vi "Udp Tester 3.vi"() -> ()   [LabVIEW 2014]
uses:
  <vilib>/addons/control/pid/pid.llb/PID EGU to Percentage (DBL).vi
  <vilib>/addons/control/pid/autopid.llb/PID Online Autotuning (Relay Feedback).vi
  <vilib>/addons/control/pid/pid.llb/PID Percentage to EGU (DBL).vi
  <vilib>/addons/control/pid/pid.llb/PID Advanced (DBL).vi
  <vilib>/FPGAPlugInAG/myRIO-1900/niLvFpga_Open_myRIO-1900.vi
  <vilib>/rvi/interface/common/dynamic/niFpgaDynamicAddResources.vi
  <vilib>/Utility/error.llb/Error Cluster From Error Code.vi
  <vilib>/rvi/errors/niLvFpgaAdjustHostInterfaceError.vi
  <vilib>/Utility/file.llb/Write To Spreadsheet File (I64).vi
  <vilib>/FPGAPlugInAG/Dynamic/niLvFpga_Close_Dynamic.vi
  <vilib>/rvi/interface/nirviOpenFPGA/nirviOpenFPGA.xnode
  FPGA Bitfiles/Test_FPGATarget_CurrentControl_60eBuCSPTsI.lvbitx
  Current Control.vi
  <vilib>/rvi/interface/nirviReadWriteControl/nirviReadWriteControl.xnode
  <vilib>/rvi/interface/nirviCloseFPGA/nirviCloseFPGA.xnode
  <vilib>/rvi/interface/Simulation/niFpgaSimulationCallBeginRW.vi
  NiFpgaLv.dll
  <vilib>/addons/control/pid/NI_PID_autopid.lvlib
  <vilib>/addons/control/pid/NI_PID_pid.lvlib
panel:
  in  "Final Output Unit":enum16{"%", "EGU"}(ring)=enum."EGU"
  in  "PID Final Min":dbl format="%.2f"
  in  "PID Final Max":dbl format="%.2f"
  in  "Intermediate Output Unit":enum16{"%", "EGU"}(ring)=enum."EGU"
  in  "Max Out":dbl format="%.2f"
  in  "Min Out":dbl format="%.2f"
  in  "Input Unit":enum16{"%", "EGU"}(ring)
  out "MV":dbl(graph)=20.39115328927357
  in  "Tab Control":enum32{"Instructions", "Plant Parameters"}(tab)
  in  "Instructions":string="Overview: This example demonstrates how to use the  PID Online Autotuning VI with the PID using the Relay Autotuning Technique.\nInstructions:\n1. Run the VI and wait until the process variable (PV) reaches near setpoint (SP).\n2.  On the PID Autotuning Design section, select the type of algorithm, type of controller and excitation amplitude for the 'open loop step response'. Then, click Autotune to start the process.\n3.  When the tuned PID gains do not change anymore or the tuning completed? flashes, the identification is done and you can accept new gains by pressing Accept gain and that will transfer the new gain to PID Gains.\n4. Click Autotune again to go back to the automatic control. You can try different options and repeat this process.\n5. Click Stop to stop the VI.\n"
  out "Plant Variable Gain":dbl=5.68817109595442
  out "Plant Variable Lag":dbl=1.4596237458843302
  in  "Load":dbl(slide) scale=0.0..10.0
  in  "Stop":bool
  out "SP and PV":cluster{"Plant Output":dbl, "SP:":dbl}(graph)
  in  "Sampling Time dt (s)":dbl=0.05 min=0.001 step=0.01 format="%#.3p"
  in  "PID Gains":T1={"proportional gain (Kc)"=0.05, "integral time (Ti, min)"=0.0, "derivative time (Td, min)"=0.0} {"derivative time (Td, min)" format="%#.6g"; "integral time (Ti, min)" format="%#.6g"; "proportional gain (Kc)" format="%#.6g"}
  in  "SP:":dbl(slide)=28.758169934640524 min=0.0 max=0.0 scale=400.0..750.0
  out "PV:":dbl(slide)=28.4408554797721 scale=400.0..750.0
  in  "Autotune":bool
  in  "Accept gain":bool
  out "tuned PID gains":T1={"proportional gain (Kc)"=1.9838195929127882, "integral time (Ti, min)"=0.01995856284686879, "derivative time (Td, min)"=0.0} {"derivative time (Td, min)" format="%#.6g"; "integral time (Ti, min)" format="%#.6g"; "proportional gain (Kc)" format="%#.6g"}
  in  "autotuning parameters":T2={"Type of Controller"=0, "relay cycles"=3, "relay amplitude"=1.0, "control specifications"=2, "PV noise level"=0.1} {"PV noise level" format="%.2f"; "control specifications" items=["fast", "normal", "slow"]; "relay amplitude" format="%.2f"; "Type of Controller" items=["P", "PI", "PID"]}
  in  "Reinitialize":bool
  in  "Automatic":bool=TRUE
  in  "alpha":dbl(slide)=0.49999999999999994 scale=0.0..1.0
  out "tuning completed?":bool
  in  "gamma":dbl(slide)=0.5102040816326531 scale=0.0..1.0
  in  "MV":dbl=60.0 format="%#_13g"
  out "error out":errorcluster
  out "Status?":bool
  out "Head Position":i32
  # "Plant Simulated Parameters"
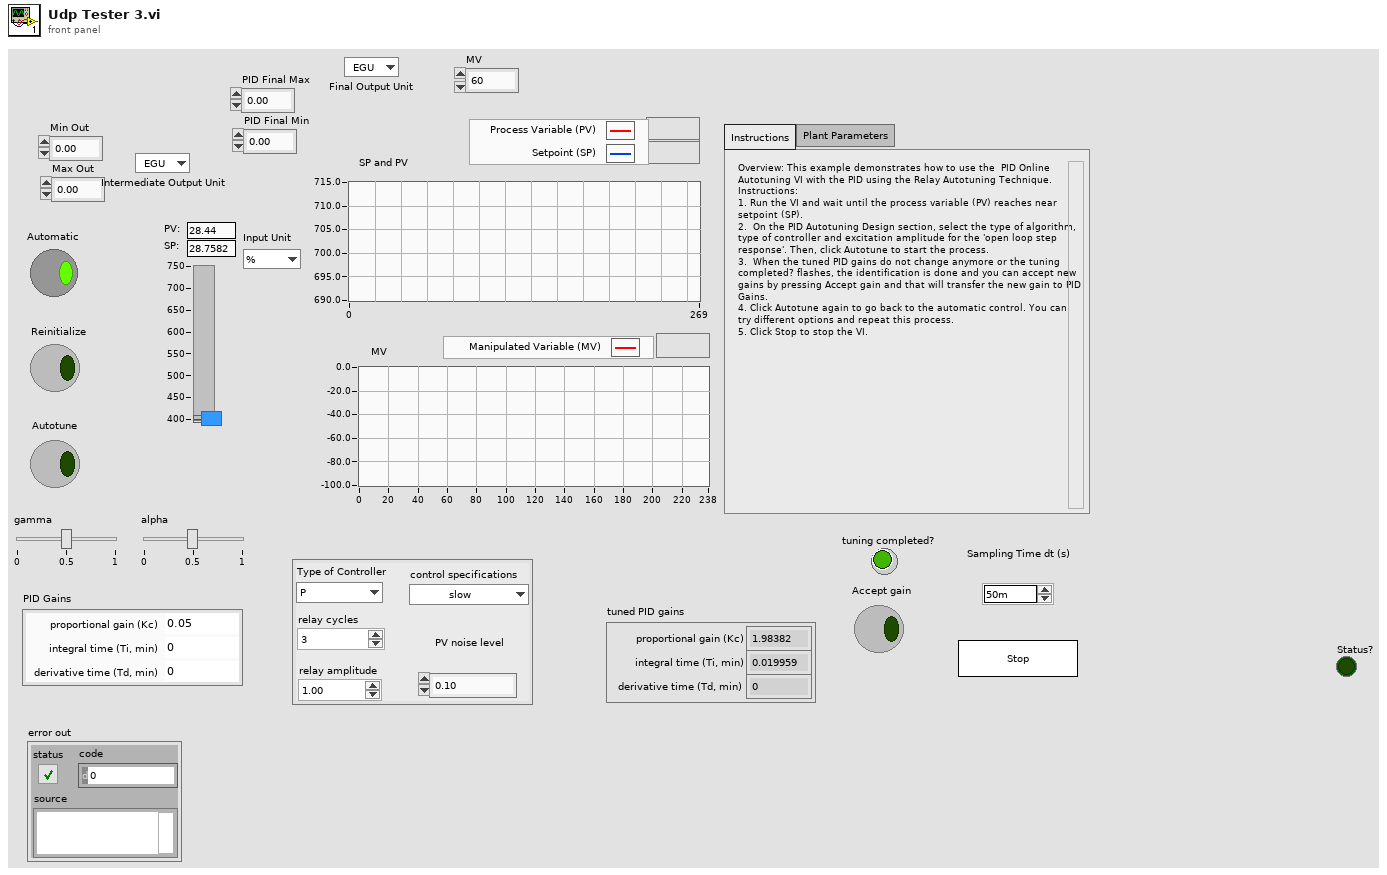
[diagram p1: front panel]
types:
  T1 = cluster{"proportional gain (Kc)":dbl, "integral time (Ti, min)":dbl, "derivative time (Td, min)":dbl}
  T2 = cluster{"Type of Controller":u16, "relay cycles":i32, "relay amplitude":dbl, "control specifications":u16, "PV noise level":dbl}
  T3 = cluster{"static gain":dbl, "lag (s)":dbl, "deadtime (s)":dbl, "load":dbl, "deadband":dbl, "sensor noise":dbl, "initial PV":dbl, "plant noise":dbl}
  T4 = enum16{"big-endian, network order", "native, host order", "little-endian"}
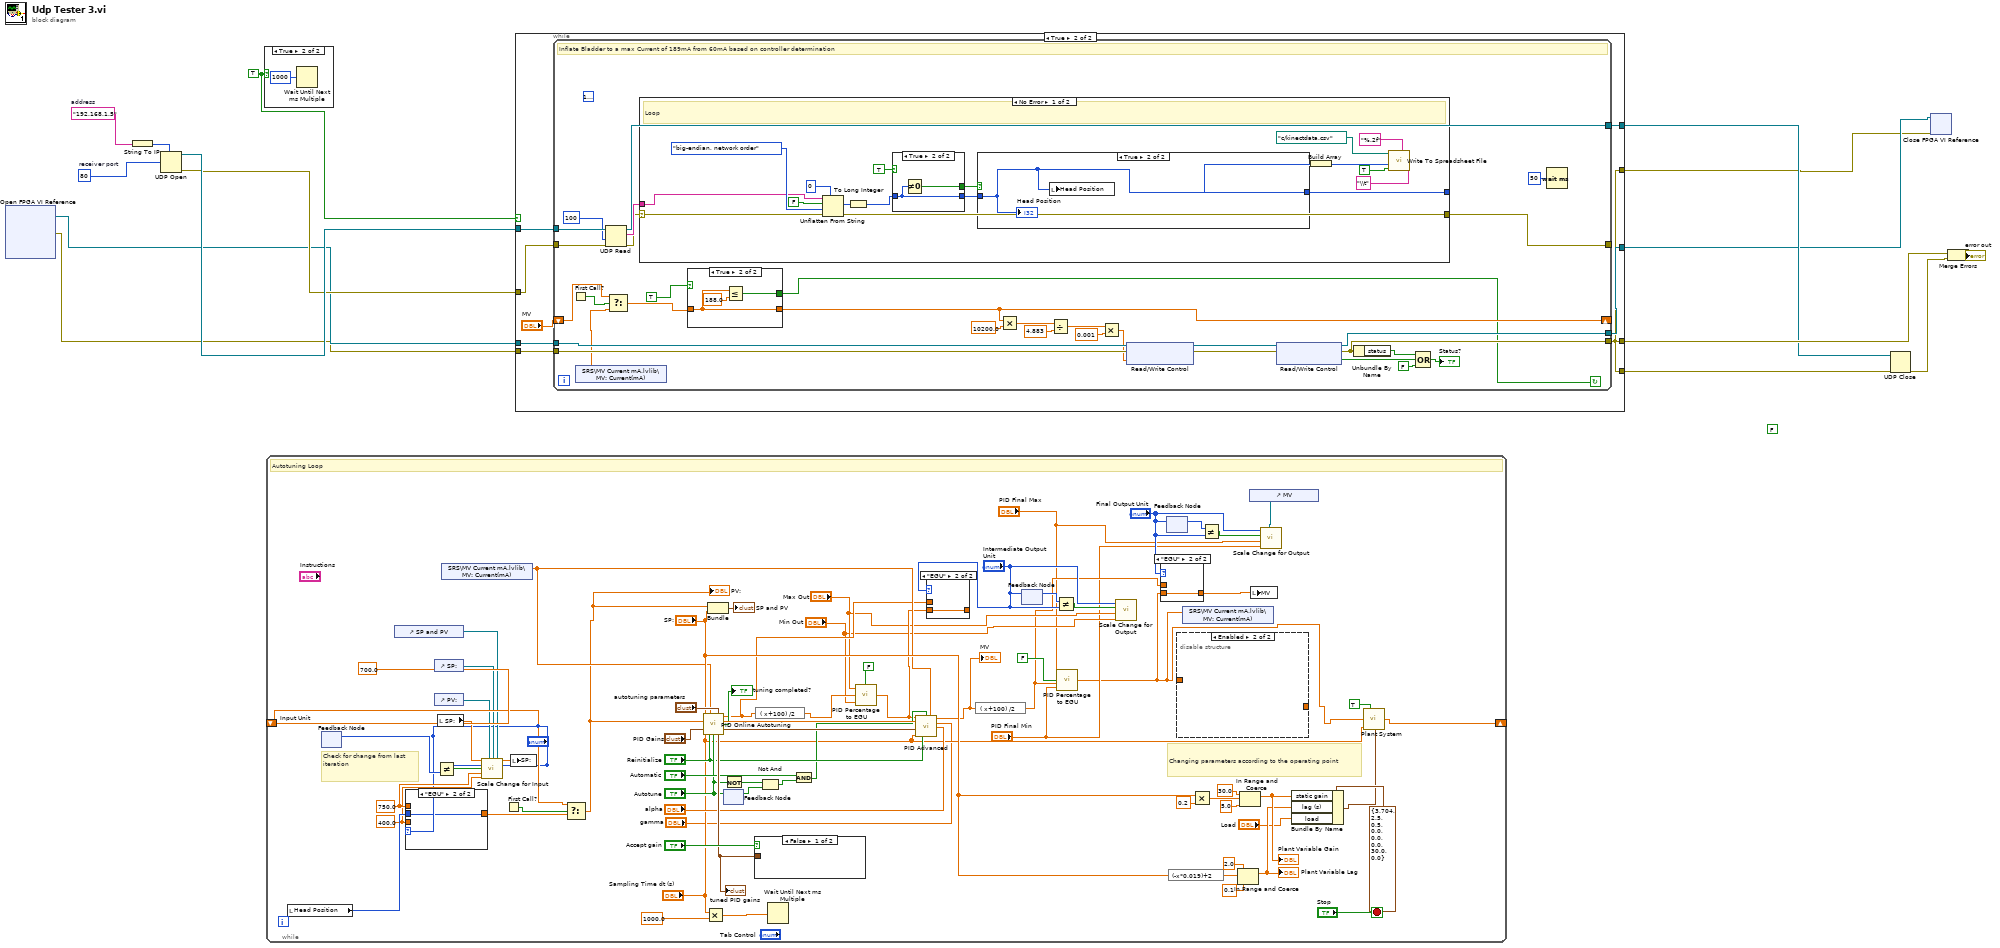
[diagram p0: block diagram]
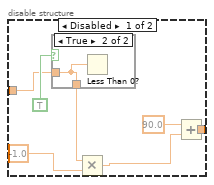
[diagram p2: hidden frame]
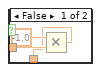
[diagram p3: hidden frame]
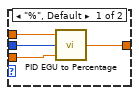
[diagram p6: hidden frame]
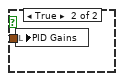
[diagram p7: hidden frame]
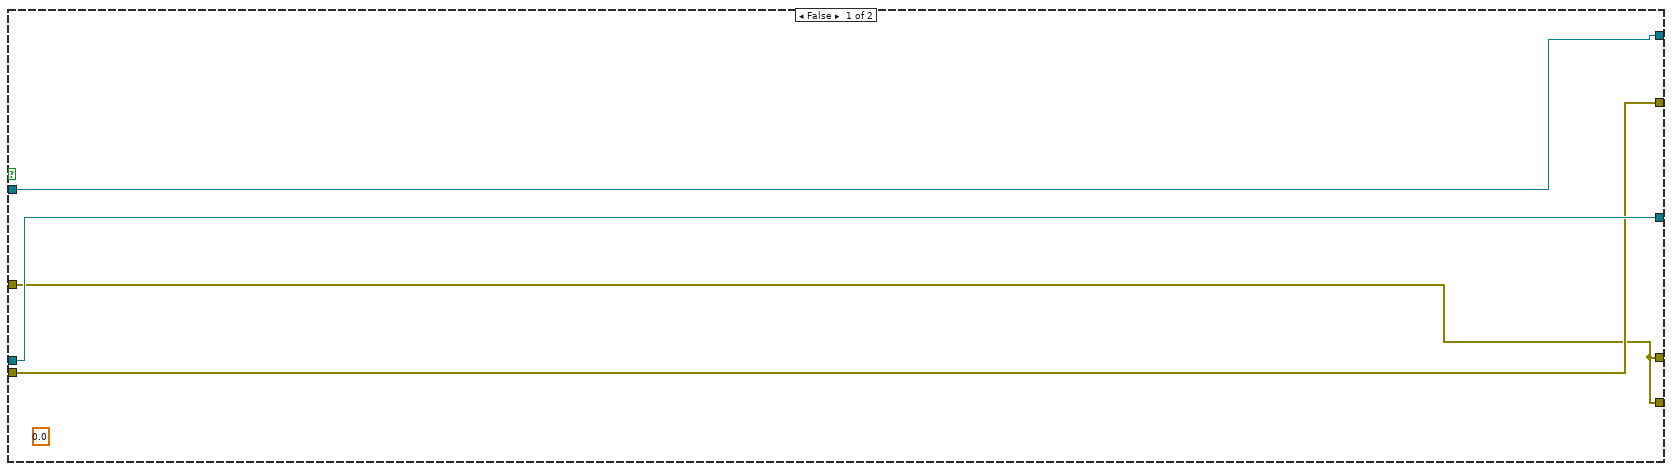
[diagram p9: hidden frame]
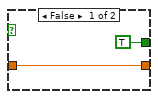
[diagram p10: hidden frame]
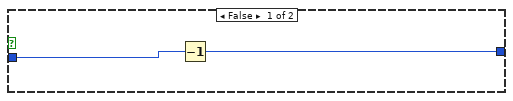
[diagram p11: hidden frame]
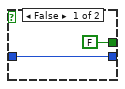
[diagram p12: hidden frame]
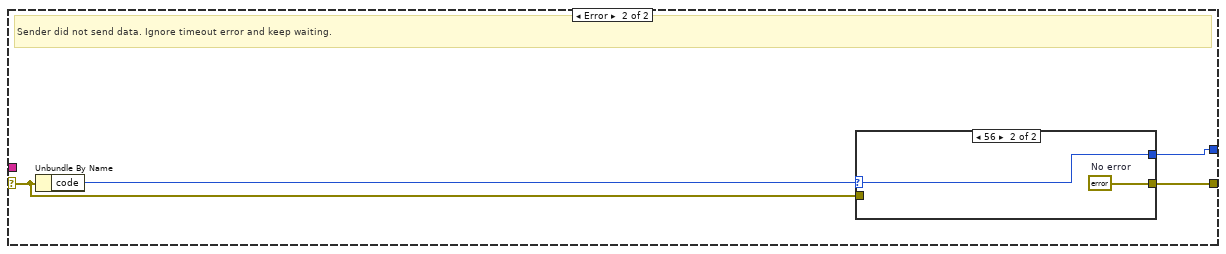
[diagram p13: hidden frame]
diagram:
  w2 = TRUE
  (unwired) FALSE
  w15 = "192.168.1.5"  # address
  w14 = u16 80  # receiver port
  n1 = xnode "Open FPGA VI Reference"() -> ("FPGA VI Reference Out"=w4:refnum<k20>, "error out"=w3:errorcluster)  [unwired: 2 in]
  n2 = String To IP(1:w15) -> (0:w16:u32)
  n3 = UDP Open(7:w16, 11:w14) -> (port=w13:refnum<k16>, 0:w12:errorcluster)  [unwired: 3 in, 1 out]
  n4 = case shown="True" w2 {
    frame False {
    }
    frame True {
      n5 = Wait Until Next ms Multiple(millisecond multiple=u32 1000) -> ()  [unwired: 1 out]
    }
  }
  n6 = while {
    shift-left: 700.0 ("Plant Output") -> [w51]
    shift-right: [w87] -> _
    stop <- "Stop" stop-if-true
    w45 = 750.0 ("Max In")
    w44 = 400.0 ("Min In")
    # "Check for change from last iteration"
    # "Changing parameters according to the operating point"
    # "Autotuning Loop"
    n7 = local read "Head Position"() -> (w49:i32)
    n8 = feedback #1() -> (w47:enum16{"%", "EGU"})  [unwired: 1 out]
    n9 = feedback-in #1("Input Unit") -> ()
    n10 = control-ref of="SP and PV"() -> (w40:refnum<vi>)
    n11 = case shown="\"EGU\"" "Input Unit" {
      tunnel: w49 -> [w108 w109]
      tunnel: [w107 w109] -> w48
      tunnel: w45 -> [w106 _]
      tunnel: w44 -> [w105 _]
      frame "%", Default {
        n12 = call-poly <vilib>:"PID EGU to Percentage.vi"("minimum (EGU)"=w105, "input (EGU)"=w108, "maximum (EGU)"=w106) -> ("% span"=w107:dbl)
      }
      frame "EGU" {
      }
    }
    n13 = control-ref of="SP:"() -> (w39:refnum<vi>)
    n14 = control-ref of="PV:"() -> (w41:refnum<vi>)
    n15 = Not Equal?(x="Input Unit", y=w47) -> (x != y?=w46:bool)
    n16 = local read "SP:"() -> (w42:dbl)
    n17 = shared-variable "SRS\\MV Current mA.lvlib\\MV: Current(mA)"() -> (w53:dbl)  [unwired: 1 in, 1 out]
    n18 = call "Scale Change for Input.vi"("SP:"=w42, "Slide Refnum"=w41, "Slide Refnum 2"=w39, "WFChart Refnum"=w40, "Input Unit"="Input Unit", "Change Scales"=w46, "Max In"=w45, "Min In"=w44) -> ("SP After Scale Change"=w43:dbl)  [unwired: 3 in, 4 out]
    n19 = First Call?() -> (First Call?: T/F=w52:bool)
    n20 = local write "SP:"(w43) -> ()
    n21 = Select(t=w51, s=w52, f=w48) -> (s? t:f=w50:dbl)
    "PV:" <- w50
    n22 = call-poly <vilib>:"PID Online Autotuning.vi"("setpoint"="SP:", "manipulated variable"=w53, "autotuning parameters"="autotuning parameters", "process variable"=w50, "PID gains in"="PID Gains", "dt (s)"="Sampling Time dt (s)", "reinitialize? (F)"="Reinitialize", "autotune? (F)"="Autotune") -> ("setpoint out"=w35:dbl, "process variable out"=w78:dbl, "tuning completed?"=→"tuning completed?":bool, "PID gains out"=w74:T1, "tuned PID gains"=w73:T1)  [unwired: 3 in]
    "tuned PID gains" <- w73
    n23 = Multiply(x="Sampling Time dt (s)", y=1000.0) -> (x*y=w55:dbl)
    n24 = Bundle("% span"=w50, "SP:"="SP:") -> (→"SP and PV":cluster{"% span":dbl, "SP:":dbl})  [unwired: 1 in]
    n25 = feedback #2() -> (w71:bool)  [unwired: 1 in]
    n26 = feedback-in #2("Autotune") -> ()
    n27 = Not(x="Autotune") -> (.not. x?=w68:bool)
    n28 = case shown="False" "Accept gain" {
      tunnel: w73 -> [_ w110]
      frame False {
      }
      frame True {
        n29 = local write "PID Gains"(w110) -> ()
      }
    }
    n30 = expression code="( x+100) /2"(w35) -> (w37:dbl)
    n31 = Not And(1:w71, 2:w68) -> (0:w69:bool)
    n32 = Wait Until Next ms Multiple(millisecond multiple=w55) -> ()  [unwired: 1 out]
    n33 = And(x="Automatic", y=w69) -> (x .and. y?=w58:bool)
    n34 = call-poly <vilib>:"PID Percentage to EGU.vi"("coerce output to range? (T)"=FALSE, "minimum (EGU)"="Min Out", "% span"=w37, "maximum (EGU)"="Max Out") -> ("output (EGU)"=w34:dbl)
    n35 = call-poly <vilib>:"PID Advanced.vi"("setpoint"=w34, "auto? (T)"=w58, "manual control"=w53, "process variable"=w78, "gamma"="gamma", "alpha"="alpha", "PID gains"=w74, "dt (s)"="Sampling Time dt (s)", "reinitialize? (F)"="Reinitialize") -> ("output"=w20:dbl)  [unwired: 5 in, 1 out]
    "MV" <- w20
    n36 = case shown="\"EGU\"" "Intermediate Output Unit" {
      tunnel: w35 -> [w103 _]
      tunnel: [w103 w104] -> _
      tunnel: w34 -> [_ w104]
      frame "%", Default {
      }
      frame "EGU" {
      }
    }
    n37 = expression code="( x+100) /2"(w20) -> (w23:dbl)
    n38 = feedback #3() -> (w33:enum16{"%", "EGU"})  [unwired: 1 out]
    n39 = feedback-in #3("Intermediate Output Unit") -> ()
    n40 = Not Equal?(x=w33, y="Intermediate Output Unit") -> (x != y?=w32:bool)
    n41 = call-poly <vilib>:"PID Percentage to EGU.vi"("coerce output to range? (T)"=FALSE, "minimum (EGU)"="PID Final Min", "% span"=w23, "maximum (EGU)"="PID Final Max") -> ("output (EGU)"=w18:dbl)
    n42 = call "Scale Change for Output.vi"("Min Out"="Min Out", "Max Out"="Max Out", "Boolean"=w32, "Output Unit"="Intermediate Output Unit") -> ()  [unwired: 6 in, 2 out]
    n43 = case shown="\"EGU\"" "Final Output Unit" {
      tunnel: w23 -> [w101 _]
      tunnel: [w101 w102] -> w24
      tunnel: w18 -> [_ w102]
      frame "%", Default {
      }
      frame "EGU" {
      }
    }
    n44 = feedback #4() -> (w27:enum16{"%", "EGU"})  [unwired: 1 out]
    n45 = feedback-in #4("Final Output Unit") -> ()
    n46 = expression code="(-x*0.019)+2"("SP:") -> (w79:dbl)
    n47 = disable-structure shown="Enabled" {
      disable-tunnel: [w93 _] -> _
      disable-tunnel: _ -> [w90 _]
      frame Disabled {
        n48 = case shown="True" TRUE {
          tunnel: w90 -> [w99 w100]
          tunnel: [w97 w100] -> w95
          frame False {
            n49 = Multiply(x=-1.0, y=w99) -> (x*y=w97:dbl)
          }
          frame True {
            n50 = Less Than 0?(x=w100) -> ()  [unwired: 1 out]
          }
        }
        n51 = Multiply(x=w95, y=-1.0) -> (x*y=w92:dbl)
        n52 = Add(x=90.0, y=w92) -> (x+y=w93:dbl)
      }
      frame Enabled {
      }
    }
    n53 = shared-variable "SRS\\MV Current mA.lvlib\\MV: Current(mA)"(w18) -> ()  [unwired: 1 in, 1 out]
    n54 = Multiply(x="SP:", y=0.2) -> (x*y=w83:dbl)
    n55 = Not Equal?(x=w27, y="Final Output Unit") -> (x != y?=w25:bool)
    n56 = In Range and Coerce(upper limit=2.0, x=w79, lower limit=0.1) -> (coerced(x)=w63:dbl)  [unwired: 1 out]
    "Plant Variable Lag" <- w63
    n57 = In Range and Coerce(upper limit=30.0, x=w83, lower limit=5.0) -> (coerced(x)=w64:dbl)  [unwired: 1 out]
    "Plant Variable Gain" <- w64
    n58 = control-ref of="MV"() -> (w19:refnum<vi>)
    n59 = local write "MV"(w24) -> ()
    n60 = call "Scale Change for Output.vi"("WFChart Refnum"=w19, "Min Out"="PID Final Min", "Max Out"="PID Final Max", "Boolean"=w25, "Output Unit"="Final Output Unit") -> ()  [unwired: 5 in, 2 out]
    n61 = Bundle By Name(cluster=T3 {"static gain"=3.704, "lag (s)"=2.5, "deadtime (s)"=0.5, "load"=0.0, "deadband"=0.0, "sensor noise"=0.0, "initial PV"=30.0, "plant noise"=0.0} ("process parameters"), "static gain"=w64, "lag (s)"=w63, "load"="Load") -> (w54:T3)
    n62 = call "Plant System.vi"("Integrator ?"=TRUE, "Plant Input"=w18, "dt (s)"="Sampling Time dt (s)", "process parameters"=w54) -> ("Plant Output"=w87:dbl)  [unwired: 11 in]
  }
  n63 = case shown="True" w2 {
    tunnel: w13 -> [w114 w122]
    tunnel: w12 -> [w111 w121]
    tunnel: [w111 w116] -> w11
    tunnel: [w114 w120] -> w10
    tunnel: [w111 w116] -> w9
    tunnel: w3 -> [w112 w119]
    tunnel: w4 -> [w113 w118]
    tunnel: [w113 w117] -> w6
    tunnel: [w112 w116] -> w5
    frame False {
      (unwired) 0.0
    }
    frame True {
      n64 = while {
        tunnel: w122 -> [w153]
        tunnel: w121 -> [w152]
        tunnel: w118 -> [w147]
        tunnel: [w148] -> w117
        tunnel: w119 -> [w150]
        tunnel: [w149] -> w116
        tunnel: [w132] -> _
        tunnel: [w131] -> w120
        shift-right: [w128] -> _
        shift-left: "MV" -> [w125]
        stop <- w127 continue-if-true
        (unwired) u32 16777216
        # "Inflate Bladder to a max Current of 189mA from 60mA based on controller determination"
        n65 = First Call?() -> (First Call?: T/F=w126:bool)
        n66 = shared-variable "SRS\\MV Current mA.lvlib\\MV: Current(mA)"() -> (w123:dbl)  [unwired: 1 in, 1 out]
        n67 = UDP Read(connection ID=w153, timeout ms (25000)=100, 8:w152) -> (data out=w134:string, error out=w133:errorcluster, 3:w131:refnum<k16>)  [unwired: 3 out]
        n68 = Select(t=w125, s=w126, f=w123) -> (s? t:f=w124:dbl)
        n69 = case shown="No Error" w133 {
          selector: w133 -> [w170 w185]
          tunnel: w134 -> [w171 _]
          tunnel: [w169 w184] -> w132
          tunnel: [w160 w183] -> _
          frame No Error {
            # "Loop"
            n70 = Unflatten From String(type=0, binary string=w171, data includes array or string size? (T)=FALSE, byte order (0:big-endian, network order)=T4."big-endian, network order" ("byte order"), error in (no error)=w170) -> (value=w172:i32, error out=w169:errorcluster)  [unwired: 1 out]
            n71 = To Long Integer(number=w172) -> (32bit integer=w167:i32)
            n72 = case shown="True" TRUE {
              tunnel: w167 -> [w179 w181]
              tunnel: [FALSE w182] -> w166
              tunnel: [w179 w181] -> w159
              frame False {
              }
              frame True {
                n73 = Not Equal To 0?(x=w181) -> (x != 0?=w182:bool)
              }
            }
            n74 = case shown="True" w166 {
              tunnel: w159 -> [w177 w178]
              tunnel: [w176 w178] -> w160
              frame False {
                n75 = Decrement(x=w177) -> (x-1=w176:i32)
              }
              frame True {
                n76 = local write "Head Position"(w178) -> ()
                "Head Position" <- w178
              }
            }
            n77 = Build Array(w160) -> (w165:i32[])
            n78 = call-poly <vilib>:"Write To Spreadsheet File.vi"("delimiter (\\t)"="\\t" ("delimiter (\\t)"), "format (%d)"="%.2f", "append to file? (new file:F)"=TRUE, "1D data"=w165, "file path (dialog if empty)"=path "c:/kinectdata.csv") -> ()  [unwired: 3 in, 1 out]
          }
          frame Error {
            # "Sender did not send data. Ignore timeout error and keep waiting."
            n79 = Unbundle By Name(w185) -> ("code"=w186:i32)
            n80 = case shown="56" w186 {
              selector: w186 -> [w187 w189]
              tunnel: w185 -> [w188 _]
              tunnel: [w188 w190] -> w184
              tunnel: [w187 w189] -> w183
              frame Default {
              }
              frame 56 {
                w190 = errorcluster {"status"=FALSE, "code"=0, "source"=""}  # No error
              }
            }
          }
        }
        n81 = case shown="True" TRUE {
          tunnel: w124 -> [w155 w156]
          tunnel: [TRUE w157] -> w127
          tunnel: [w155 w156] -> w128
          frame False {
          }
          frame True {
            n82 = Less Or Equal?(x=w156, y=188.0) -> (x <= y?=w157:bool)
          }
        }
        n83 = Multiply(x=w128, y=10200.0) -> (x*y=w135:dbl)
        n84 = Divide(x=w135, y=4.883) -> (x/y=w138:dbl)
        n85 = Multiply(x=w138, y=0.001) -> (x*y=w144:dbl)
        n86 = xnode "Read/Write Control"("FPGA VI Reference In"=w147, "error in"=w150, "DAC Inlet Valve"=w144) -> ("FPGA VI Reference Out"=w146:refnum<k20>, "error out"=w145:errorcluster)
        n87 = xnode "Read/Write Control"("FPGA VI Reference In"=w146, "error in"=w145) -> ("FPGA VI Reference Out"=w148:refnum<k20>, "error out"=w149:errorcluster, "Inlet Overflow?"=w143:bool)
        n88 = Unbundle By Name(w149) -> ("status"=w141:bool)
        n89 = Compound Arithmetic op=OR(w141, w143, FALSE ("value")) -> (→"Status?":bool)
        n90 = Wait (ms)(milliseconds to wait=u32 50) -> ()  [unwired: 1 out]
      }
    }
  }
  n91 = UDP Close(connection ID=w10, 8:w9) -> (error out=w8:errorcluster)  [unwired: 1 out]
  n92 = xnode "Close FPGA VI Reference"("FPGA VI Reference In"=w6, "error in"=w5) -> ()  [unwired: 1 out]
  n93 = Merge Errors(w11, w8) -> (→"error out":errorcluster)
